vi "axex_get_sheet_ref.vi"(8 "error in":errorcluster, 11 "AX Excel instance in":T1) -> (0 "error out":errorcluster, 1 "sheet name":string, 2 "sheet ref out":refnum<k7>, 3 "AX Excel instance out":T1)   [LabVIEW 2020, in "AX Excel.lvlib"]
doc: "Call this to get reference of the selected sheet (selected sheet: sheet selected by 'sxe_select_sheet.vi'). If no sheet was selected yet an active sheet reference will be returned (active sheet: the sheet that is visible in M$ Excel).\n\nDon't close the reference, it remains opened in SX Excel instance handle until another sheet is selected or excel is closed!"
uses:
  AX Excel.lvlib
  axex_instance.ctl
  <vilib>/Utility/error.llb/Error Cluster From Error Code.vi
  <vilib>/ErrorRing/Error Ring.xnode
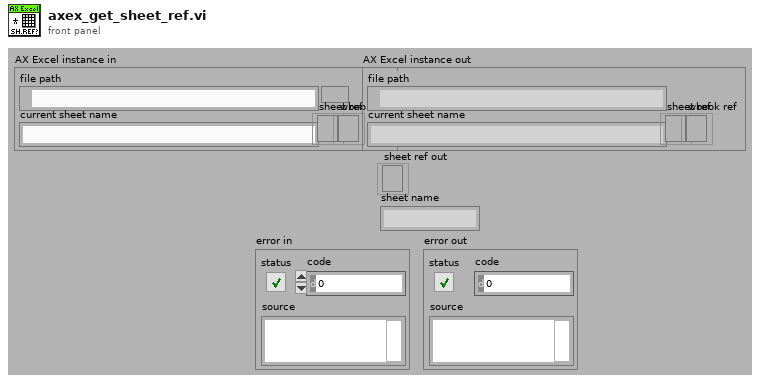
[diagram p1: front panel]
types:
  T1 = typedef "AX Excel.lvlib/axex_instance.ctl" = cluster{"file path":path, "current sheet name":string, "sheet ref":refnum<k7>, "wbook ref":refnum<k7>}
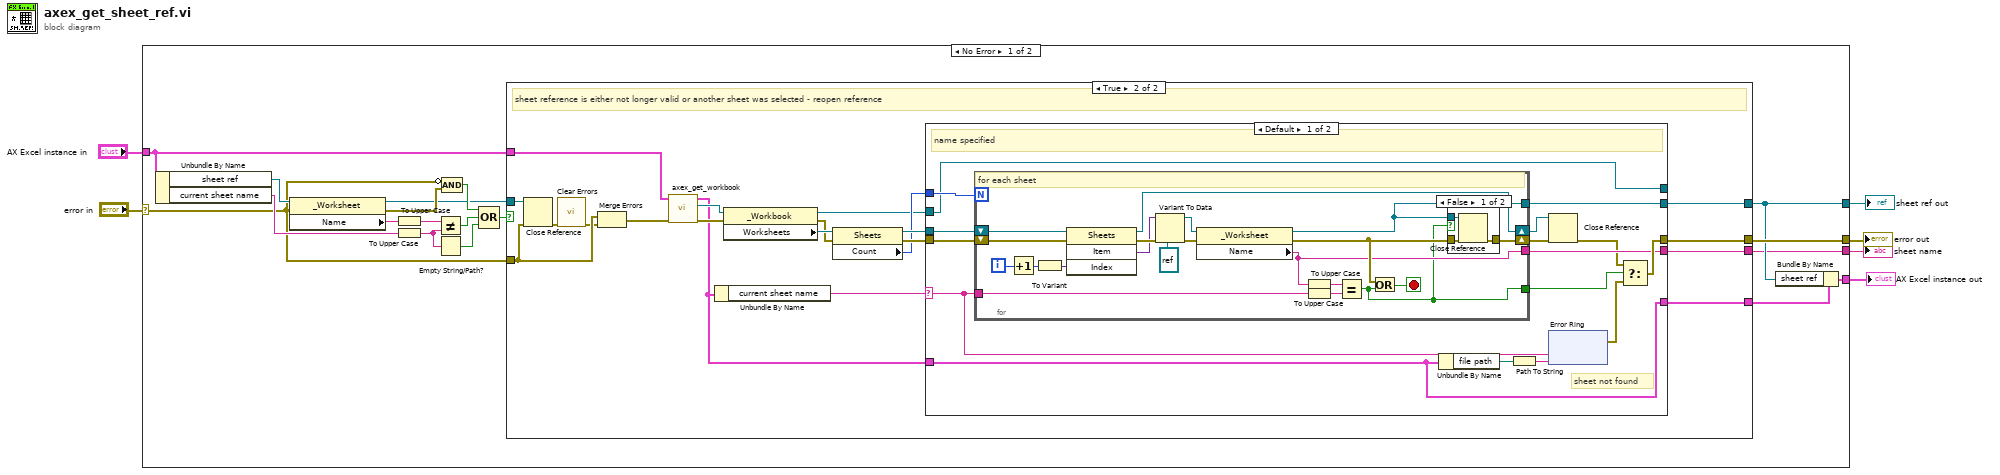
[diagram p0: block diagram]
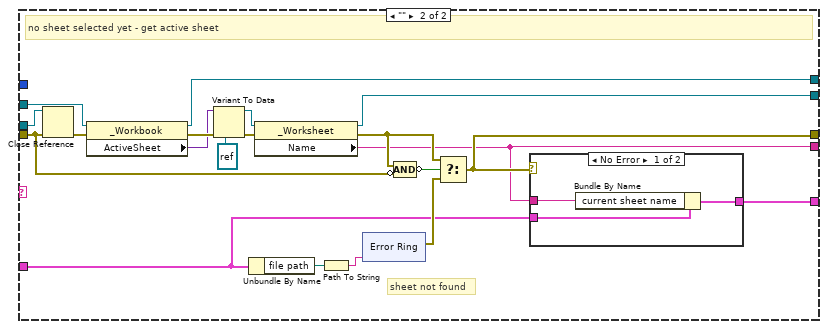
[diagram p4: hidden frame]
diagram:
  n1 = case shown="No Error" "error in" {
    selector: "error in" -> [w7 w128]
    tunnel: "AX Excel instance in" -> [w17 w127]
    tunnel: [w14 w128] -> w5
    tunnel: [w12 _] -> w4
    tunnel: [w11 w127] -> w3
    tunnel: [w8 _] -> w2
    frame No Error {
      n2 = Unbundle By Name(w17) -> ("sheet ref"=w24:refnum<k7>, "current sheet name"=w15:string)
      n3 = property class="_Worksheet"(reference=w24, error in=w7) -> (reference out=w19:refnum<k7>, error out=w22:errorcluster, "Name"=w23:string)
      n4 = To Upper Case(1:w23) -> (0:w10:string)
      n5 = To Upper Case(1:w15) -> (0:w9:string)
      n6 = Not Equal?(x=w10, y=w9) -> (x != y?=w21:bool)
      n7 = Empty String/Path?(string/path=w9) -> (empty?=w16:bool)
      n8 = Compound Arithmetic op=AND(invert w7, w22) -> (w20:bool)
      n9 = Compound Arithmetic op=OR(w20, w21, w16) -> (w18:bool)
      n10 = case shown="True" w18 {
        tunnel: [w27 w29] -> w14
        tunnel: [w26 w47] -> w13
        tunnel: [w25 w46] -> w12
        tunnel: w7 -> [w27 w45]
        tunnel: w19 -> [w25 w44]
        tunnel: w17 -> [w26 w30]
        tunnel: [_ w28] -> w8
        frame False {
          # "sheet reference is still valid and sheet name matches current sheet"
        }
        frame True {
          # "sheet reference is either not longer valid or another sheet was selected - reopen reference"
          n11 = Close Reference(reference=w44, error in (no error)=w45) -> (error out=w43:errorcluster)
          n12 = call <vilib>:"Clear Errors.vi"("error in (no error)"=w43) -> ("error out"=w42:errorcluster)  [unwired: 5 in, 1 out]
          n13 = Merge Errors(w45, w42) -> (w41:errorcluster)
          n14 = call "axex_get_workbook.vi"("error in"=w41, "AX Excel instance in"=w30) -> ("error out"=w40:errorcluster, "excel workbook"=w34:refnum<k7>, "AX Excel instance out"=w31:T1)  [unwired: 7 in]
          n15 = Unbundle By Name(w31) -> ("current sheet name"=w33:string)
          n16 = property class="_Workbook"(reference=w34, error in=w40) -> (reference out=w32:refnum<k7>, error out=w38:errorcluster, "Worksheets"=w39:refnum<k7>)
          n17 = property class="Sheets"(reference=w39, error in=w38) -> (reference out=w37:refnum<k7>, error out=w36:errorcluster, "Count"=w35:i32)
          n18 = case shown="Default" w33 {
            selector: w33 -> [w56 _]
            tunnel: w37 -> [w63 w114]
            tunnel: w36 -> [w62 w104]
            tunnel: w35 -> [w61 _]
            tunnel: [w57 w99] -> w29
            tunnel: [w60 w102] -> w46
            tunnel: [w54 w97] -> w28
            tunnel: w32 -> [w53 w113]
            tunnel: [w53 w106] -> _
            tunnel: w31 -> [w48 w98]
            tunnel: [w48 w96] -> w47
            frame Default {
              # "sheet not found"
              # "name specified"
              n19 = for {
                N: w61 -> [_]
                shift-right: [w84] -> w52
                shift-left: w62 -> [w88]
                shift-right: [w86] -> w51
                shift-left: w63 -> [w87]
                tunnel: w56 -> [w85]
                tunnel: [w74] -> w59
                tunnel: [w82] -> w60
                tunnel: [w80] -> w54
                i -> [w89]
                stop <- w81 stop-if-true
                # "for each sheet"
                n20 = Increment(x=w89) -> (x+1=w90:i32)
                n21 = To Variant(anything=w90) -> (Variant=w91:variant)
                n22 = invoke class="Sheets" method="Item"(reference=w87, error in=w88, "Index"=w91) -> (reference out=w86:refnum<k7>, error out=w78:errorcluster, "Item"=w76:variant)  [unwired: 1 in, 1 out]
                n23 = Variant To Data(error in=w78, type=refnum<k7> refnum ("reference out"), Variant=w76) -> (data=w75:refnum<k7>, error out=w77:errorcluster)
                n24 = property class="_Worksheet"(reference=w75, error in=w77) -> (reference out=w82:refnum<k7>, error out=w83:errorcluster, "Name"=w80:string)
                n25 = To Upper Case(1:w80) -> (0:w73:string)
                n26 = To Upper Case(1:w85) -> (0:w72:string)
                n27 = Equal?(x=w73, y=w72) -> (x = y?=w74:bool)
                n28 = Or(x=w83, y=w74) -> (x .or. y?=w81:bool)
                n29 = case shown="False" w74 {
                  tunnel: [w94 w95] -> w84
                  tunnel: w83 -> [w93 w95]
                  tunnel: w82 -> [w92 _]
                  frame False {
                    n30 = Close Reference(reference=w92, error in (no error)=w93) -> (error out=w94:errorcluster)
                  }
                  frame True {
                  }
                }
              }
              n31 = Unbundle By Name(w48) -> ("file path"=w49:path)
              n32 = Path To String(path=w49) -> (string=w55:string)
              n33 = Close Reference(reference=w51, error in (no error)=w52) -> (error out=w50:errorcluster)
              n34 = xnode "Error Ring"("parameter 0"=w56, "parameter 1"=w55) -> ("error out"=w58:errorcluster)
              n35 = Select(t=w50, s=w59, f=w58) -> (s? t:f=w57:errorcluster)
            }
            frame "" {
              # "sheet not found"
              # "no sheet selected yet - get active sheet"
              n36 = Close Reference(reference=w114, error in (no error)=w104) -> (error out=w112:errorcluster)
              n37 = property class="_Workbook"(reference=w113, error in=w112) -> (reference out=w106:refnum<k7>, error out=w110:errorcluster, "ActiveSheet"=w109:variant)
              n38 = Variant To Data(error in=w110, type=refnum<k7> refnum ("reference out"), Variant=w109) -> (data=w107:refnum<k7>, error out=w108:errorcluster)
              n39 = Unbundle By Name(w98) -> ("file path"=w100:path)
              n40 = property class="_Worksheet"(reference=w107, error in=w108) -> (reference out=w102:refnum<k7>, error out=w103:errorcluster, "Name"=w97:string)
              n41 = Path To String(path=w100) -> (string=w101:string)
              n42 = xnode "Error Ring"("parameter 0"=w101) -> ("error out"=w115:errorcluster)
              n43 = Compound Arithmetic op=AND(w103, invert w104) -> (invert w105:bool)
              n44 = Select(t=w103, s=w105, f=w115) -> (s? t:f=w99:errorcluster)
              n45 = case shown="No Error" w99 {
                tunnel: w98 -> [w118 w119]
                tunnel: w97 -> [w117 _]
                tunnel: [w116 w119] -> w96
                frame No Error {
                  n46 = Bundle By Name(cluster=w118, "current sheet name"=w117) -> (w116:T1)
                }
                frame Error {
                }
              }
            }
          }
        }
      }
      n47 = Bundle By Name(cluster=w13, "sheet ref"=w12) -> (w11:T1)
    }
    frame Error {
    }
  }
  "error out" <- w5
  "AX Excel instance out" <- w3
  "sheet ref out" <- w4
  "sheet name" <- w2
